vi "index_four_axes.vi"(8 "x_index":i32, 11 "graph_data":cluster{"array type (2D Dbl)":dbl[], dbl[]}[](array[cluster])) -> (0 "Y4":dbl, 1 "Y3":dbl, 2 "Y2":dbl, 3 "Y1":dbl, 5 "X":dbl)   [LabVIEW 2025]
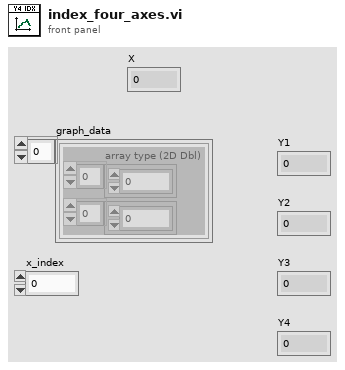
[diagram p1: front panel]
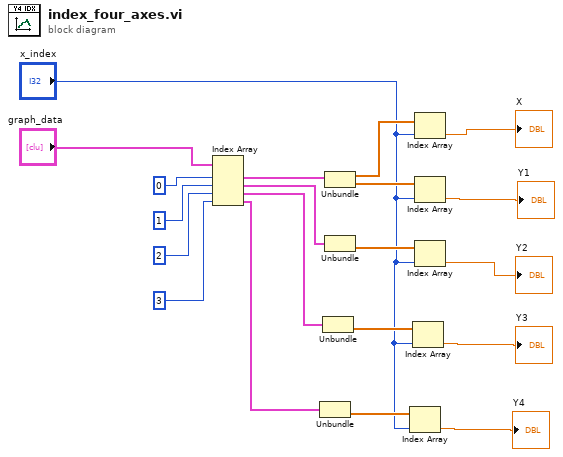
[diagram p0: block diagram]
diagram:
  n1 = Index Array(array="graph_data", index #1=0 ("index"), index #2=1 ("index"), index #3=2 ("index"), index #4=3 ("index")) -> (element #1=w14:cluster{"array type (2D Dbl)":dbl[], dbl[]}, element #2=w11:cluster{"array type (2D Dbl)":dbl[], dbl[]}, element #3=w6:cluster{"array type (2D Dbl)":dbl[], dbl[]}, element #4=w2:cluster{"array type (2D Dbl)":dbl[], dbl[]})
  n2 = Unbundle(w2) -> (w4:dbl[])  [unwired: 1 out]
  n3 = Unbundle(w6) -> (w8:dbl[])  [unwired: 1 out]
  n4 = Unbundle(w14) -> ("array type (2D Dbl)"=w16:dbl[], w13:dbl[])
  n5 = Unbundle(w11) -> (w12:dbl[])  [unwired: 1 out]
  n6 = Index Array(array=w4, index="x_index") -> (element=→"Y4":dbl)
  n7 = Index Array(array=w8, index="x_index") -> (element=→"Y3":dbl)
  n8 = Index Array(array=w16, index="x_index") -> (element=→"X":dbl)
  n9 = Index Array(array=w13, index="x_index") -> (element=→"Y1":dbl)
  n10 = Index Array(array=w12, index="x_index") -> (element=→"Y2":dbl)
